vi "Cell Enable.vi"(7 "Box ID":u8, 8 "error in (no error)":errorcluster, 9 "Enable":bool, 10 "Channel":u16=1 min=1 max=12 step=1, 11 "ENET in":refnum<class "ENET_BS120x.lvclass">) -> (0 "error out":errorcluster, 3 "ENET out":refnum<class "ENET_BS120x.lvclass">)   [LabVIEW 2021, in "BS120x Driver.lvlib" / "ENET_BS120x.lvclass"]
uses:
  ENET_BS120x.lvclass
  BS120x.lvclass
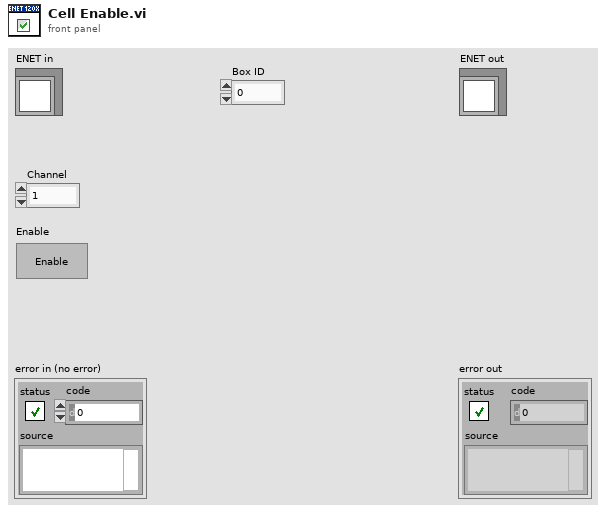
[diagram p1: front panel]
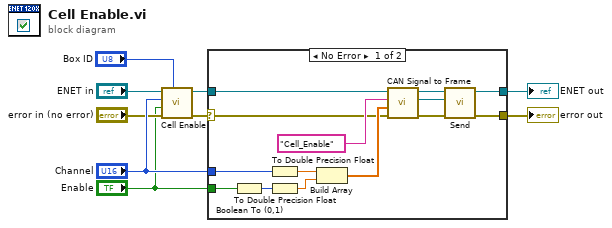
[diagram p0: block diagram]
diagram:
  n1 = call-parent "Cell Enable.vi"("Box ID"="Box ID", "error in (no error)"="error in (no error)", "Enable"="Enable", "Channel"="Channel", "BS120x in"="ENET in") -> ("error out"=w3:errorcluster, "BS120x out"=w6:refnum<class "ENET_BS120x.lvclass">)  [unwired: 5 in]
  n2 = case shown="No Error" w3 {
    selector: w3 -> [w10 w24]
    tunnel: [w19 w24] -> w9
    tunnel: "Enable" -> [w15 _]
    tunnel: [w13 w25] -> w8
    tunnel: w6 -> [w12 w25]
    tunnel: "Channel" -> [w11 _]
    frame No Error {
      n3 = Boolean To (0,1)(Boolean=w15) -> (0, 1=w16:i16)
      n4 = To Double Precision Float(number=w11) -> (double precision float=w18:dbl)
      n5 = To Double Precision Float(number=w16) -> (double precision float=w17:dbl)
      n6 = Build Array(w18, w17) -> (w14:dbl[])
      n7 = call "CAN Signal to Frame.vi"("error in (no error)"=w10, "Data Array"=w14, "Frame"="Cell_Enable", "ENET in"=w12) -> ("error out"=w20:errorcluster, "Data"=w21:refnum<class "Data.lvclass">, "ENET out"=w22:refnum<class "ENET_BS120x.lvclass">)  [unwired: 5 in]
      n8 = call "Send.vi"("error in (no error)"=w20, "Data"=w21, "ENET in"=w22) -> ("error out"=w19:errorcluster, "ENET out"=w13:refnum<class "ENET_BS120x.lvclass">)  [unwired: 7 in]
    }
    frame Error {
    }
  }
  "error out" <- w9
  "ENET out" <- w8
